vi "Create Dir in FTP if Not Exist.vi"(8 "error in (no error)":errorcluster, 10 "dir":string, 11 "FTPProtocol in":refnum<class "FTPProtocol.lvclass">) -> (0 "error out":errorcluster, 3 "FTPProtocol out":refnum<class "FTPProtocol.lvclass">)   [LabVIEW 2020, in "FileSync -- FTP.lvlib" / "FTPProtocol.lvclass"]
uses:
  FTPProtocol.lvclass
  FTPProtocol.lvclass/FTPProtocol.ctl
  Read FTP.vi
  <userlib>/_OpenG.lib/array/array.llb/Filter 1D Array with Scalar (String)__ogtk.vi
  _support/FTP Toolkit/FTP Class/FTP.lvclass
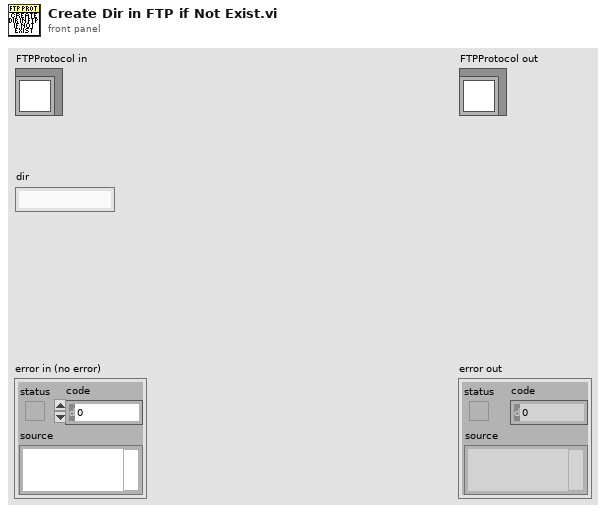
[diagram p1: front panel]
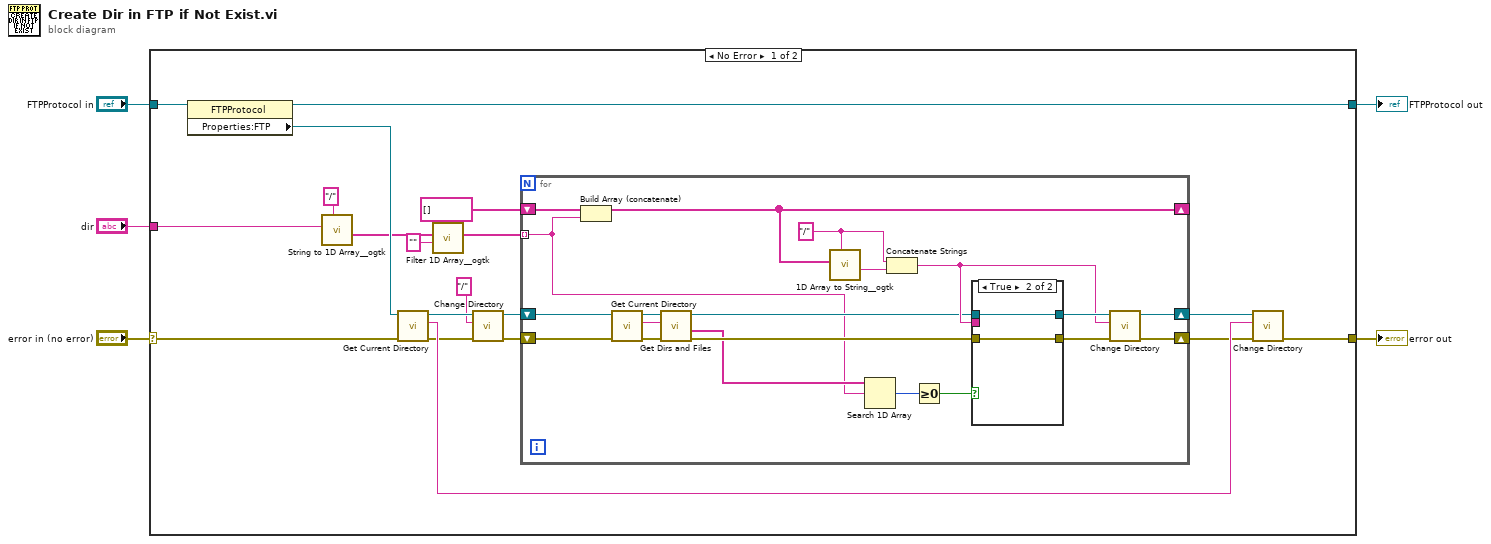
[diagram p0: block diagram]
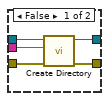
[diagram p2: hidden frame]
diagram:
  n1 = case shown="No Error" "error in (no error)" {
    selector: "error in (no error)" -> [w14 w53]
    tunnel: [w17 w53] -> w4
    tunnel: [w23 w52] -> w2
    tunnel: "FTPProtocol in" -> [w24 w52]
    tunnel: "dir" -> [w21 _]
    frame No Error {
      n2 = property class="FTPProtocol"(reference=w24) -> (reference out=w23:refnum<class "FTPProtocol.lvclass">, "Properties:FTP"=w16:refnum<class "FTP.lvclass">)  [unwired: 1 in, 1 out]
      n3 = call <userlib>:"String to 1D Array__ogtk.vi"("delimiter (Tab)"="/", "string"=w21) -> ("Array of Strings"=w12:string[])  [unwired: 9 in]
      n4 = call "Get Current Directory.vi"("error in (no error)"=w14, "FTP in"=w16) -> ("error out"=w9:errorcluster, "Current Directory"=w19:string, "FTP out"=w10:refnum<class "FTP.lvclass">)  [unwired: 7 in]
      n5 = call-poly <userlib>:"Filter 1D Array__ogtk.vi"("items to filter"="" ("delimiter (Tab)"), "array"=w12) -> ("filtered array"=w13:string[])  [unwired: 4 in, 1 out]
      n6 = call "Change Directory.vi"("error in (no error)"=w9, "RemoteDirectory"="/" ("delimiter (Tab)"), "FTP in"=w10) -> ("error out"=w7:errorcluster, "FTP out"=w8:refnum<class "FTP.lvclass">)  [unwired: 7 in]
      n7 = for {
        shift-right: [w39] -> w20
        shift-left: w8 -> [w34]
        shift-right: [w40] -> w18
        shift-left: w7 -> [w33]
        tunnel: w13 -> [w25] mode=indexing
        shift-right: [w43] -> _
        shift-left: string[] [] ("delimiter (Tab)") -> [w44]
        w37 = "/" ("delimiter (Tab)")
        n8 = Build Array (concatenate)(w44, w25) -> (w43:string[])
        n9 = call "Get Current Directory.vi"("error in (no error)"=w33, "FTP in"=w34) -> ("error out"=w32:errorcluster, "Current Directory"=w30:string, "FTP out"=w31:refnum<class "FTP.lvclass">)  [unwired: 7 in]
        n10 = call "Get Dirs and Files.vi"("error in (no error)"=w32, "RemoteDirectory"=w30, "FTP in"=w31) -> ("error out"=w35:errorcluster, "Dirs"=w26:string[], "FTP out"=w36:refnum<class "FTP.lvclass">)  [unwired: 5 in, 1 out]
        n11 = call <userlib>:"1D Array to String__ogtk.vi"("delimiter (Tab)"=w37, "Array of Strings"=w43) -> ("delimited string"=w29:string)  [unwired: 9 in]
        n12 = Search 1D Array(1D array=w26, element=w25) -> (index of element=w28:i32)  [unwired: 1 in]
        n13 = Concatenate Strings(w37, w29) -> (w38:string)
        n14 = Greater Or Equal To 0?(x=w28) -> (x >= 0?=w27:bool)
        n15 = case shown="True" w27 {
          tunnel: [w49 w51] -> w42
          tunnel: [w48 w50] -> w41
          tunnel: w38 -> [w47 _]
          tunnel: w36 -> [w46 w51]
          tunnel: w35 -> [w45 w50]
          frame False {
            n16 = call "Create Directory.vi"("error in (no error)"=w45, "Remote Directory"=w47, "FTP in"=w46) -> ("error out"=w48:errorcluster, "FTP out"=w49:refnum<class "FTP.lvclass">)  [unwired: 7 in]
          }
          frame True {
          }
        }
        n17 = call "Change Directory.vi"("error in (no error)"=w41, "RemoteDirectory"=w38, "FTP in"=w42) -> ("error out"=w40:errorcluster, "FTP out"=w39:refnum<class "FTP.lvclass">)  [unwired: 7 in]
      }
      n18 = call "Change Directory.vi"("error in (no error)"=w18, "RemoteDirectory"=w19, "FTP in"=w20) -> ("error out"=w17:errorcluster)  [unwired: 7 in, 1 out]
    }
    frame Error {
    }
  }
  "error out" <- w4
  "FTPProtocol out" <- w2
